vi "build token URI.vi"(8 "error in (no error)":errorcluster, 11 "Oauth2.QBO in":refnum<class "Oauth2.QBO.lvclass">) -> (0 "error out":errorcluster, 1 "Headers":cluster{"header":string, "value":string}[](array[cluster]), 2 "Token Request URI":string, 3 "Oauth2.QBO":refnum<class "Oauth2.QBO.lvclass">)   [LabVIEW 2013, in "Oauth2.QBO.lvclass"]
uses:
  Oauth2.QBO.lvclass
  Oauth2/Oauth2.lvclass/Oauth2.ctl
  <vilib>/LabVIEW Open Source Project/OpenSerializer.Base64/Base64_CharSet.vi
  OAuthToken/Retrieve Element.vi
  Oauth2/Oauth2.lvclass
  <vilib>/LabVIEW Open Source Project/OpenURI/uri/URI.lvclass
  <vilib>/LabVIEW Open Source Project/OpenSerializer.Base64/Serializer.Base64.lvclass
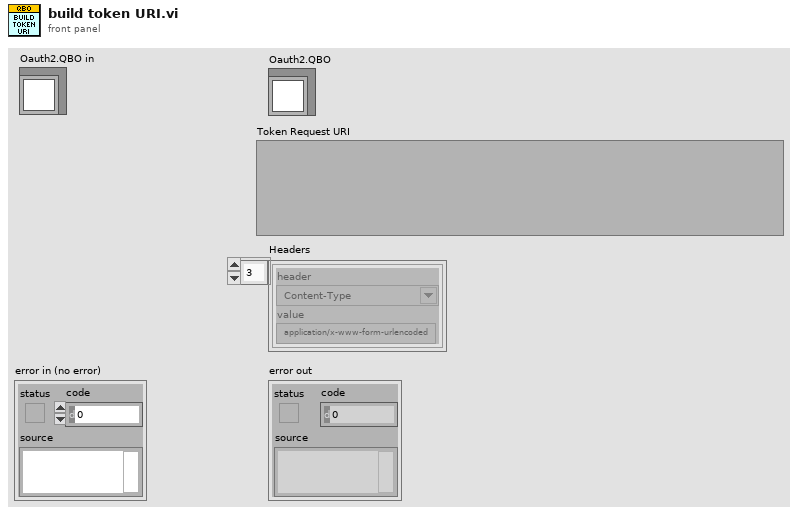
[diagram p1: front panel]
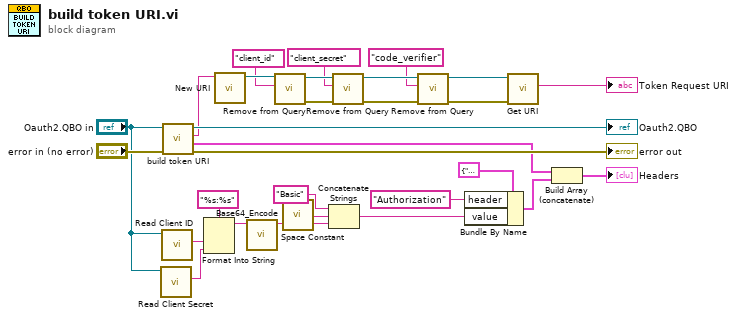
[diagram p0: block diagram]
diagram:
  n1 = call "Read Client Secret.vi"("Oauth2 in"="Oauth2.QBO in") -> ("Client Secret"=w13:string)  [unwired: 8 in, 2 out]
  n2 = call "Read Client ID.vi"("Oauth2 in"="Oauth2.QBO in") -> ("Client ID"=w14:string)  [unwired: 8 in, 2 out]
  n3 = call-parent "build token URI.vi"("error in (no error)"="error in (no error)", "Oauth2 in"="Oauth2.QBO in") -> ("error out"=→"error out":errorcluster, "Headers"=w18:cluster{"header":string, "value":string}[], "Token Request URI"=w23:string, "Oauth2"=→"Oauth2.QBO":refnum<class "Oauth2.QBO.lvclass">)  [unwired: 6 in]
  n4 = Format Into String(format string="%s:%s", w14, w13) -> (resulting string=w11:string)  [unwired: 2 in, 1 out]
  n5 = call <vilib>:"New URI.vi"("URI"=w23) -> ("URI"=w26:refnum<class "URI.lvclass">)  [unwired: 9 in, 1 out]
  n6 = call <vilib>:"Base64_Encode.vi"("String"=w11) -> ("Encoded String"=w10:string)  [unwired: 9 in, 1 out]
  n7 = call <vilib>:"Remove from Query.vi"("key"="client_id", "URI in"=w26) -> ("error out"=w21:errorcluster, "URI out"=w24:refnum<class "URI.lvclass">)  [unwired: 7 in, 1 out]
  n8 = call <vilib>:"Space Constant.vi"() -> ("String"=w7:string)
  n9 = Concatenate Strings("Basic" ("header"), w7, w10) -> (w8:string)
  n10 = call <vilib>:"Remove from Query.vi"("error in (no error)"=w21, "key"="client_secret", "URI in"=w24) -> ("error out"=w5:errorcluster, "URI out"=w3:refnum<class "URI.lvclass">)  [unwired: 6 in, 1 out]
  n11 = call <vilib>:"Remove from Query.vi"("error in (no error)"=w5, "key"="code_verifier", "URI in"=w3) -> ("error out"=w4:errorcluster, "URI out"=w2:refnum<class "URI.lvclass">)  [unwired: 6 in, 1 out]
  n12 = Bundle By Name(cluster=cluster{"header":string, "value":string} {"header"="", "value"=""} ("Header"), "header"="Authorization", "value"=w8) -> (w16:cluster{"header":string, "value":string})
  n13 = call <vilib>:"Get URI.vi"("error in (no error)"=w4, "URI in"=w2) -> ("URI String"=→"Token Request URI":string)  [unwired: 7 in, 2 out]
  n14 = Build Array (concatenate)(w18, w16) -> (→"Headers":cluster{"header":string, "value":string}[])
